vi "run.vi"(8 "error in (no error)":errorcluster, 11 "GenericExperiment in":refnum<class "ExperimentControllerDL090803Triggered.lvclass">) -> (0 "error out":errorcluster, 3 "GenericExperiment out":refnum<class "ExperimentControllerDL090803Triggered.lvclass">)   [LabVIEW 2010, in "ExperimentControllerDL090803Triggered.lvclass"]
uses:
  ExperimentControllerDL090803Triggered.lvclass
  internal_trigger_enum.ctl
  main/labview_source/controls/undock_button.ctl
  ExperimentControllerDL090803Triggered.lvclass/ExperimentControllerDL090803Triggered.ctl
  state_enum.ctl
  GenericExperimentController/GenericExperimentController/trigger_enum.ctl
  GenericExperimentController/GenericExperimentController/GenericExperimentController.lvclass
  common/classes/ErrorController/ErrorController/class_data.vi
  common/classes/ErrorController/ErrorController/ErrorController.lvclass
panel:
  in  "button:undock":T1
  in  "Tab Control":enum32{"User", "Debug", "About"}(tab)
  out "current sweep no.":i32
  out "finished?":bool
  out "last trigger":T2
  out "state chart counter":i32
  # "- With this experiment controller, each sweep is triggered by a TTL trigger to the Hifo ADC.\n- Make sure that you connect your shutter device to the Hifo ADC.\n- Check the online documentation at www.helioscan.org for details about the connectivity."
  # "ExperimentControllerDL090803Triggered"
  # "Implemented by: \nDominik Langer, University of Zurich"
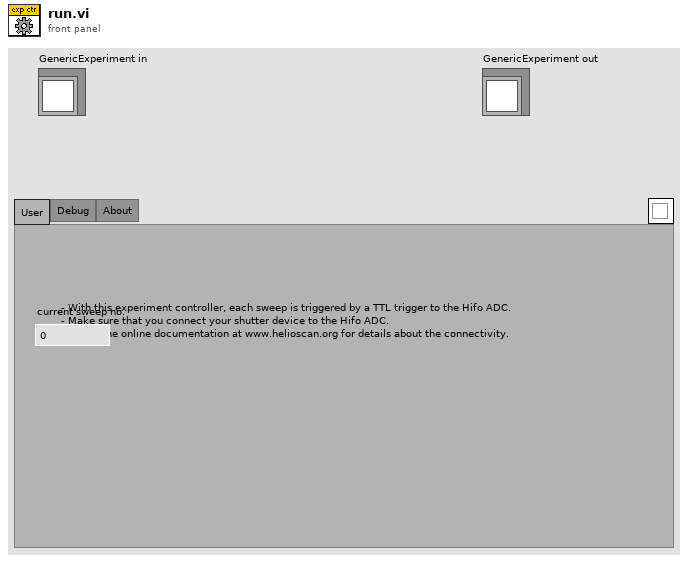
[diagram p1: front panel]
types:
  T1 = typedef "undock_button.ctl" = bool
  T2 = typedef "ExperimentControllerDL090803Triggered.lvclass/internal_trigger_enum.ctl" = enum16{"NULL", "initialise", "terminate", "proceed", "start", "stop"}
  T3 = typedef "ExperimentControllerDL090803Triggered.lvclass/state_enum.ctl" = enum16{"not in experiment", "in experiment"}
  T4 = typedef "GenericExperimentController.lvclass/trigger_enum.ctl" = enum16{"NULL", "proceed", "prepare"}
  T5 = typedef "top-level_component_type_enum.ctl" = enum16{"undefined", "ImagingMode", "ScanHead", "DAQ", "ImageAssembler", "Display", "DataCollection", "Analyser", "Stimulator", "ExperimentController", "Instrument", "Stage"}
  T6 = typedef "main_trigger_enum.ctl" = enum16{"NULL", "initialise", "terminate", "start", "stop", "change objective", "change experimentController", "change imagingMode", "save notebook", "started saving", "finished saving", "expCtr ready", "expCtr missing", "imgMd ready", "imgMd missing", "scanHd ready", "scanHd missing", "DAQ ready", "DAQ missing", "imgAsm ready", "imgAsm missing", "dataColl ready", "dataColl missing", "display ready", "display missing", "analysr ready", "analysr missing", "instrmnt ready", "instrmnt missing", "stimltr ready", "stimltr missing", "stage ready", "stage missing"}
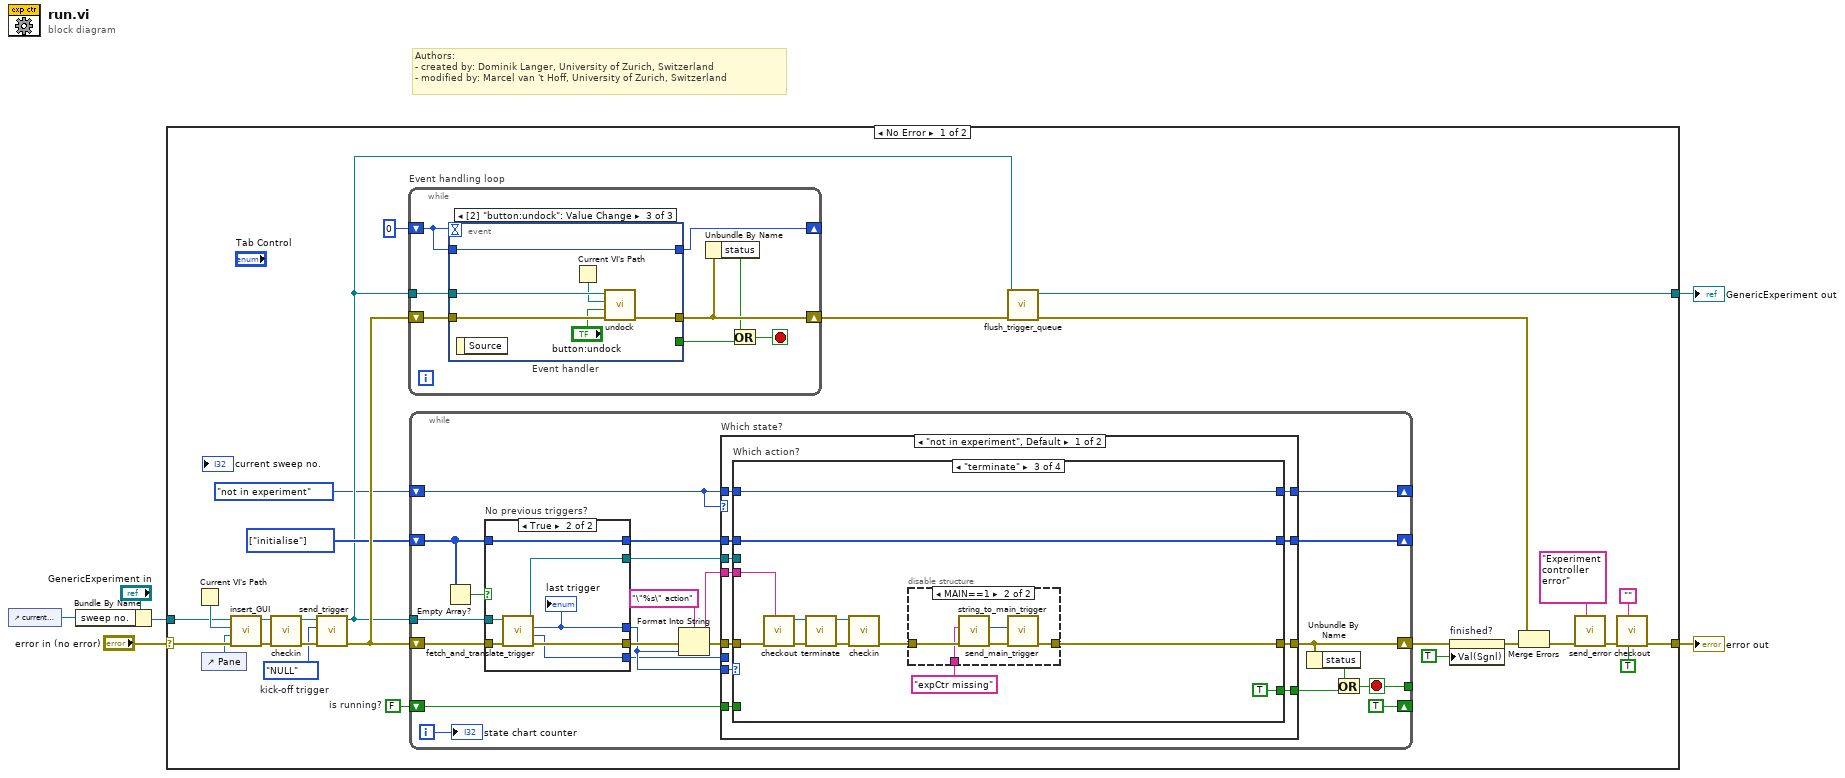
[diagram p0: block diagram]
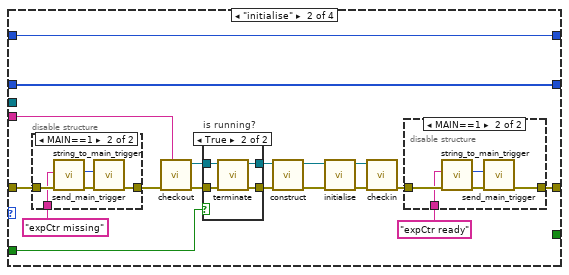
[diagram p3: hidden frame]
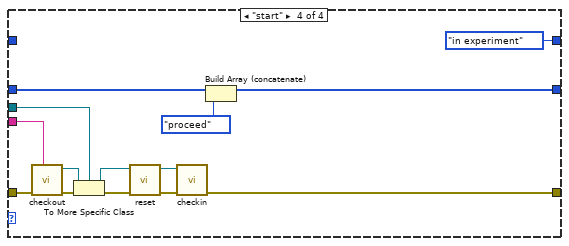
[diagram p8: hidden frame]
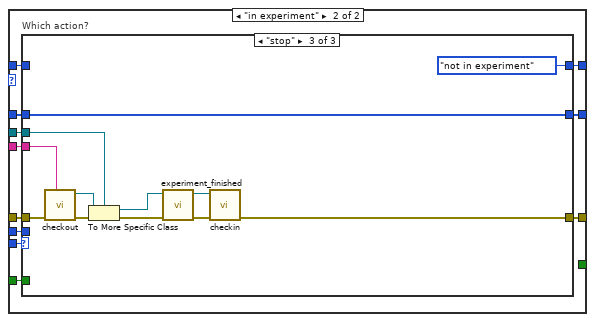
[diagram p9: hidden frame]
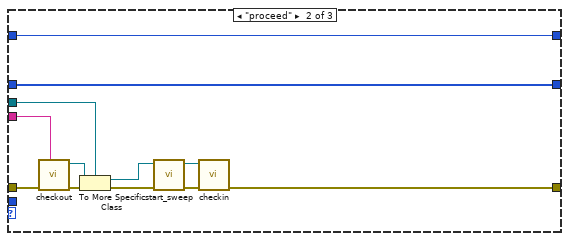
[diagram p11: hidden frame]
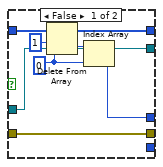
[diagram p12: hidden frame]
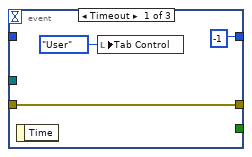
[diagram p13: hidden frame]
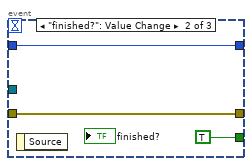
[diagram p14: hidden frame]
diagram:
  # "Authors: \n- created by: Dominik Langer, University of Zurich, Switzerland\n- modified by: Marcel van 't Hoff, University of Zurich, Switzerland"
  n1 = control-ref of="current sweep no."() -> (w1:refnum<vi>)
  n2 = Bundle By Name(cluster="GenericExperiment in", "sweep no."=w1) -> (w2:refnum<class "ExperimentControllerDL090803Triggered.lvclass">)
  n3 = case shown="No Error" "error in (no error)" {
    selector: "error in (no error)" -> [w27 w212]
    tunnel: [w32 w212] -> w5
    tunnel: [w22 w211] -> w4
    tunnel: w2 -> [w24 w211]
    frame No Error {
      w14 = FALSE  # is running?
      w15 = T2[] [enum."initialise"] items=["NULL", "initialise", "terminate", "proceed", "start", "stop"]
      w20 = trigger_enum."NULL"  # kick-off trigger
      n4 = Current VI's Path() -> (path=w26:path)
      n5 = control-ref of="Pane"() -> (w25:refnum<vi>)
      n6 = call-dynamic "insert_GUI.vi"("error in (no error)"=w27, "Pane"=w25, "VI path"=w26, "GenericComponent in"=w24) -> ("error out"=w19:errorcluster, "GenericComponent out"=w18:refnum<class "ExperimentControllerDL090803Triggered.lvclass">)  [unwired: 6 in]
      n7 = call-dynamic "checkin.vi"("error in (no error)"=w19, "GenericExperimentController in"=w18) -> ("error out"=w21:errorcluster, "GenericExperimentController out"=w17:refnum<class "ExperimentControllerDL090803Triggered.lvclass">)  [unwired: 8 in]
      n8 = call-dynamic "send_trigger.vi"("error in (no error)"=w21, "trigger"=w20, "GenericExperiment in"=w17) -> ("error out"=w16:errorcluster, "GenericExperiment out"=w13:refnum<class "ExperimentControllerDL090803Triggered.lvclass">)  [unwired: 7 in]
      n9 = while "Event handling loop" {
        shift-right: [w197] -> _
        shift-left: 0 -> [w198]
        shift-right: [w195] -> w11
        shift-left: w16 -> [w196]
        tunnel: w13 -> [w191]
        stop <- w192 stop-if-true
        n10 = event "Event handler" shown="[2] \"button:undock\": Value Change" {
          selector: _ -> [_ _ _]
          dyn-events: _ -> [_ _ _]
          timeout: w198 -> [_ _ _]
          tunnel: [-1 w204 w210] -> w197
          tunnel: w198 -> [_ w204 w210]
          tunnel: w196 -> [w200 w202 w209]
          tunnel: [w200 w202 w208] -> w195
          tunnel: [_ TRUE _] -> w193
          tunnel: w191 -> [_ _ w207]
          event Timeout {
            n11 = event-data() -> ()  [unwired: 2 out]
            n12 = local write "Tab Control"(enum32{"User", "Debug", "About"}."User" ("Tab Control")) -> ()
          }
          event "finished?": Value Change {
            n13 = event-data() -> ()  [unwired: 2 out]
          }
          event Value Change {
            n14 = event-data() -> ()  [unwired: 2 out]
            n15 = Current VI's Path() -> (path=w205:path)
            n16 = call-dynamic "undock.vi"("error in (no error)"=w209, "undock?"="button:undock", "VI path"=w205, "GenericComponent in"=w207) -> ("error out"=w208:errorcluster)  [unwired: 6 in, 1 out]
          }
        }
        n17 = Unbundle By Name(w195) -> ("status"=w194:bool)
        n18 = Or(x=w194, y=w193) -> (x .or. y?=w192:bool)
      }
      n19 = while {
        shift-right: [w40] -> w12
        shift-left: w16 -> [w55]
        shift-right: [w46] -> _
        shift-left: w15 -> [w52]
        shift-right: [TRUE ("is running?")] -> _
        shift-left: w14 -> [w43]
        tunnel: w13 -> [w54]
        tunnel: [w37] -> _
        shift-right: [w35] -> _
        shift-left: state_enum."not in experiment" ("state") -> [w34]
        i -> [w36]
        stop <- w37 stop-if-true
        n20 = Empty Array?(array=w52) -> (empty?=w53:bool)
        n21 = case "No previous triggers?" shown="True" w53 {
          tunnel: w54 -> [w183 w188]
          tunnel: w55 -> [w181 w189]
          tunnel: [w183 w187] -> w47
          tunnel: [w179 w184] -> w49
          tunnel: [_ w185] -> w41
          tunnel: [w181 w186] -> w50
          tunnel: w52 -> [w182 w190]
          tunnel: [w178 w190] -> w45
          frame False {
            w176 = 0 ("index")
            n22 = Delete From Array(array=w182, length=1, index=w176) -> (deleted portion=w180:T2[], array with subset deleted=w178:T2[])
            n23 = Index Array(array=w180, index=w176) -> (element=w179:T2)
          }
          frame True {
            n24 = call-dynamic "fetch_and_translate_trigger.vi"("error in (no error)"=w189, "ExperimentControllerDL090803Triggered in"=w188) -> ("error out"=w186:errorcluster, "sender TLC type"=w185:T5, "statechart trigger"=w184:T2, "ExperimentControllerDL090803Triggered out"=w187:refnum<class "ExperimentControllerDL090803Triggered.lvclass">)  [unwired: 6 in]
            "last trigger" <- w184
          }
        }
        n25 = Format Into String(format string="\"%s\" action", error in=w50, w49) -> (resulting string=w44:string, error out=w48:errorcluster)  [unwired: 1 in]
        n26 = case "Which state?" shown="\"not in experiment\", Default" w34 {
          tunnel: w49 -> [w57 w148]
          tunnel: w48 -> [w58 w147]
          tunnel: w47 -> [w62 w146]
          tunnel: [w65 w145] -> w46
          tunnel: w45 -> [w63 w144]
          tunnel: w44 -> [w61 w143]
          tunnel: w43 -> [w56 w142]
          tunnel: w41 -> [_ w141]
          tunnel: [w59 w140] -> w40
          tunnel: [w60 _] -> w39
          tunnel: w34 -> [w64 w139]
          tunnel: [w66 w138] -> w35
          frame "not in experiment", Default {
            n27 = case "Which action?" shown="\"terminate\"" w57 {
              tunnel: [w68 w73 w108 w128] -> w59
              tunnel: w58 -> [w68 w86 w111 w131]
              tunnel: w62 -> [_ _ _ w129]
              tunnel: [w69 w87 w117 w126] -> w65
              tunnel: w63 -> [w69 w87 w117 w127]
              tunnel: w61 -> [_ w80 w110 w130]
              tunnel: w56 -> [_ w79 _ _]
              tunnel: [_ _ TRUE _] -> w60
              tunnel: w64 -> [w67 w72 w107 _]
              tunnel: [w67 w72 w107 state_enum."in experiment" ("state")] -> w66
              frame "NULL", Default {
              }
              frame "initialise" {
                n28 = disable-structure shown="MAIN==1" {
                  disable-tunnel: [w100 w105] -> w81
                  disable-tunnel: w86 -> [w100 w104]
                  disable-tunnel: "expCtr missing" -> [_ w101]
                  frame condition #0 {
                  }
                  frame condition #1 (active) {
                    n29 = call "string_to_main_trigger.vi"("error in (no error)"=w104, "trigger string"=w101) -> ("error out"=w103:errorcluster, "main trigger"=w102:T6)  [unwired: 8 in]
                    n30 = call "send_main_trigger.vi"("error in (no error)"=w103, "trigger"=w102) -> ("error out"=w105:errorcluster)  [unwired: 9 in]
                  }
                }
                n31 = call "checkout.vi"("locked by?"=w80, "error in (no error)"=w81) -> ("error out"=w78:errorcluster, "GenericExperimentController out"=w77:refnum<class "GenericExperimentController.lvclass">)  [unwired: 1 in, 7 out]
                n32 = case "is running?" shown="True" w79 {
                  tunnel: w78 -> [w95 w99]
                  tunnel: w77 -> [w94 w98]
                  tunnel: [w95 w96] -> w76
                  tunnel: [w94 w97] -> w75
                  frame False {
                  }
                  frame True {
                    n33 = call-dynamic "terminate.vi"("error in (no error)"=w99, "GenericPlugin in"=w98) -> ("error out"=w96:errorcluster, "GenericPlugin out"=w97:refnum<class "GenericExperimentController.lvclass">)  [unwired: 8 out]
                  }
                }
                n34 = call-dynamic "construct.vi"("error in (no error)"=w76, "GenericPlugin in"=w75) -> ("error out"=w82:errorcluster, "GenericPlugin out"=w83:refnum<class "GenericExperimentController.lvclass">)  [unwired: 2 in, 6 out]
                n35 = call-dynamic "initialise.vi"("error in (no error)"=w82, "GenericPlugin in"=w83) -> ("error out"=w84:errorcluster, "GenericPlugin out"=w85:refnum<class "GenericExperimentController.lvclass">)  [unwired: 8 out]
                n36 = call-dynamic "checkin.vi"("error in (no error)"=w84, "GenericExperimentController in"=w85) -> ("error out"=w74:errorcluster)  [unwired: 8 in, 1 out]
                n37 = disable-structure shown="MAIN==1" {
                  disable-tunnel: [w88 w93] -> w73
                  disable-tunnel: w74 -> [w88 w92]
                  disable-tunnel: "expCtr ready" -> [_ w89]
                  frame condition #0 {
                  }
                  frame condition #1 (active) {
                    n38 = call "string_to_main_trigger.vi"("error in (no error)"=w92, "trigger string"=w89) -> ("error out"=w91:errorcluster, "main trigger"=w90:T6)  [unwired: 8 in]
                    n39 = call "send_main_trigger.vi"("error in (no error)"=w91, "trigger"=w90) -> ("error out"=w93:errorcluster)  [unwired: 9 in]
                  }
                }
              }
              frame "terminate" {
                n40 = call "checkout.vi"("locked by?"=w110, "error in (no error)"=w111) -> ("error out"=w112:errorcluster, "GenericExperimentController out"=w113:refnum<class "GenericExperimentController.lvclass">)  [unwired: 1 in, 7 out]
                n41 = call-dynamic "terminate.vi"("error in (no error)"=w112, "GenericPlugin in"=w113) -> ("error out"=w114:errorcluster, "GenericPlugin out"=w115:refnum<class "GenericExperimentController.lvclass">)  [unwired: 8 out]
                n42 = call-dynamic "checkin.vi"("error in (no error)"=w114, "GenericExperimentController in"=w115) -> ("error out"=w109:errorcluster)  [unwired: 8 in, 1 out]
                n43 = disable-structure shown="MAIN==1" {
                  disable-tunnel: [w118 w123] -> w108
                  disable-tunnel: w109 -> [w118 w121]
                  disable-tunnel: "expCtr missing" -> [_ w119]
                  frame condition #0 {
                  }
                  frame condition #1 (active) {
                    n44 = call "string_to_main_trigger.vi"("error in (no error)"=w121, "trigger string"=w119) -> ("error out"=w120:errorcluster, "main trigger"=w122:T6)  [unwired: 8 in]
                    n45 = call "send_main_trigger.vi"("error in (no error)"=w120, "trigger"=w122) -> ("error out"=w123:errorcluster)  [unwired: 9 in]
                  }
                }
              }
              frame "start" {
                n46 = call "checkout.vi"("locked by?"=w130, "error in (no error)"=w131) -> ("error out"=w134:errorcluster, "GenericExperimentController out"=w135:refnum<class "GenericExperimentController.lvclass">)  [unwired: 1 in, 7 out]
                n47 = To More Specific Class(target class=w129, reference=w135, error in=w134) -> (specific class reference=w136:refnum<class "ExperimentControllerDL090803Triggered.lvclass">, error out=w133:errorcluster)
                n48 = call-dynamic "reset.vi"("error in (no error)"=w133, "DL090430TriggeredExperimentController in"=w136) -> ("error out"=w132:errorcluster, "DL090430TriggeredExperimentController out"=w137:refnum<class "ExperimentControllerDL090803Triggered.lvclass">)  [unwired: 8 out]
                n49 = call-dynamic "checkin.vi"("error in (no error)"=w132, "GenericExperimentController in"=w137) -> ("error out"=w128:errorcluster)  [unwired: 8 in, 1 out]
                n50 = Build Array (concatenate)(w127, internal_trigger_enum."proceed" ("Enum")) -> (w126:T2[])
              }
            }
          }
          frame "in experiment" {
            n51 = case "Which action?" shown="\"stop\"" w148 {
              tunnel: [w150 w153 w167] -> w140
              tunnel: w147 -> [w150 w156 w168]
              tunnel: w146 -> [_ w154 w166]
              tunnel: [w151 w163 w175] -> w145
              tunnel: w144 -> [w151 w163 w175]
              tunnel: w143 -> [_ w155 w165]
              tunnel: w142 -> [_ _ _]
              tunnel: w141 -> [_ _ _]
              tunnel: w139 -> [w149 w152 _]
              tunnel: [w149 w152 state_enum."not in experiment" ("state")] -> w138
              frame "NULL", Default {
              }
              frame "proceed" {
                n52 = call "checkout.vi"("locked by?"=w155, "error in (no error)"=w156) -> ("error out"=w157:errorcluster, "GenericExperimentController out"=w158:refnum<class "GenericExperimentController.lvclass">)  [unwired: 1 in, 7 out]
                n53 = To More Specific Class(target class=w154, reference=w158, error in=w157) -> (specific class reference=w160:refnum<class "ExperimentControllerDL090803Triggered.lvclass">, error out=w159:errorcluster)
                n54 = call-dynamic "start_sweep.vi"("error in (no error)"=w159, "DL090430TriggeredExperimentController in"=w160) -> ("error out"=w161:errorcluster, "DL090430TriggeredExperimentController out"=w162:refnum<class "ExperimentControllerDL090803Triggered.lvclass">)  [unwired: 8 out]
                n55 = call-dynamic "checkin.vi"("error in (no error)"=w161, "GenericExperimentController in"=w162) -> ("error out"=w153:errorcluster)  [unwired: 8 in, 1 out]
              }
              frame "stop" {
                n56 = call "checkout.vi"("locked by?"=w165, "error in (no error)"=w168) -> ("error out"=w169:errorcluster, "GenericExperimentController out"=w170:refnum<class "GenericExperimentController.lvclass">)  [unwired: 1 in, 7 out]
                n57 = To More Specific Class(target class=w166, reference=w170, error in=w169) -> (specific class reference=w172:refnum<class "ExperimentControllerDL090803Triggered.lvclass">, error out=w171:errorcluster)
                n58 = call-dynamic "experiment_finished.vi"("error in (no error)"=w171, "DL090430TriggeredExperimentController in"=w172) -> ("error out"=w173:errorcluster, "DL090430TriggeredExperimentController out"=w174:refnum<class "ExperimentControllerDL090803Triggered.lvclass">)  [unwired: 8 out]
                n59 = call-dynamic "checkin.vi"("error in (no error)"=w173, "GenericExperimentController in"=w174) -> ("error out"=w167:errorcluster)  [unwired: 8 in, 1 out]
              }
            }
          }
        }
        n60 = Unbundle By Name(w40) -> ("status"=w38:bool)
        n61 = Or(x=w38, y=w39) -> (x .or. y?=w37:bool)
        "state chart counter" <- w36
      }
      n62 = call-dynamic "flush_trigger_queue.vi"("error in (no error)"=w11, "GenericToplevelComponent in"=w13) -> ("error out"=w23:errorcluster, "GenericToplevelComponent out"=w22:refnum<class "ExperimentControllerDL090803Triggered.lvclass">)  [unwired: 8 in]
      n63 = property on="finished?" class="Bool (strict)"(error in=w12, "Val(Sgnl)"=TRUE) -> (error out=w30:errorcluster)  [unwired: 1 in, 1 out]
      n64 = Merge Errors(w23, w30) -> (w10:errorcluster)
      n65 = call "send_error.vi"("additional message"="Experiment controller error", "error in (no error)"=w10) -> ("error out"=w9:errorcluster)  [unwired: 9 in]
      n66 = call "checkout.vi"("destroy queue?"=TRUE, "locked by?"="", "error in (no error)"=w9) -> ("error out"=w32:errorcluster)  [unwired: 8 out]
    }
    frame Error {
    }
  }
  "error out" <- w5
  "GenericExperiment out" <- w4
